vi "CRCgenerator.vi"(1 "String":string="this is a test string") -> (0 "CRC-16-CCITT-0xFFFF":u16 format="%.0x")   [LabVIEW 2012]
uses:
  CRC SubVIs/Wrappers/CRC-16-CCITT-0xFFFF.vi
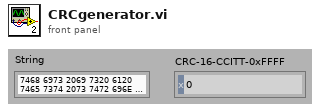
[diagram p1: front panel]
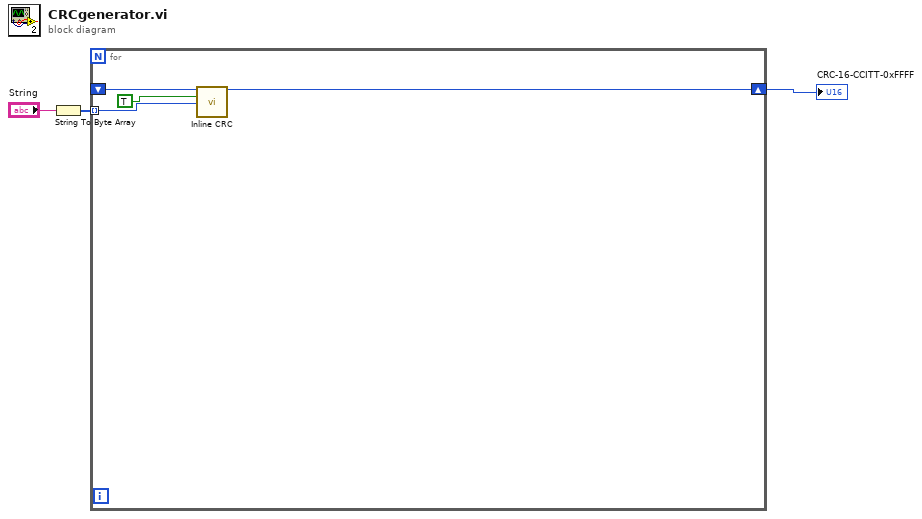
[diagram p0: block diagram]
diagram:
  n1 = String To Byte Array(string="String") -> (unsigned byte array=w2:u8[])
  n2 = for {
    shift-right: [w7] -> w1
    shift-left: _ -> [w6]
    tunnel: w2 -> [w5] mode=indexing
    n3 = call-poly "Inline CRC.vi"("CRC In"=w6, "Reset"=TRUE, "Data"=w5) -> ("CRC"=w7:u16)  [unwired: 11 in, 1 out]
  }
  "CRC-16-CCITT-0xFFFF" <- w1
